vi "TriggererBoolean.vi"(8 "Boolean":bool, 10 "Control Name":string="Acquire Trigger", 11 "name or relative path":string="SW-Microscoper.vi") -> (0 "error out":errorcluster, 3 "VI out":refnum<vi>)   [LabVIEW 2012]
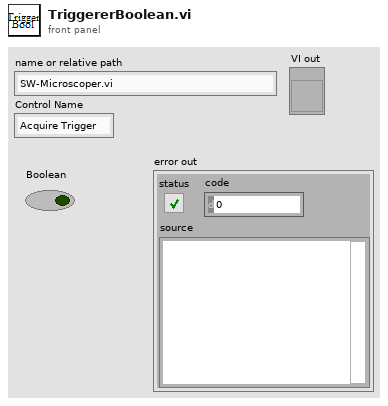
[diagram p1: front panel]
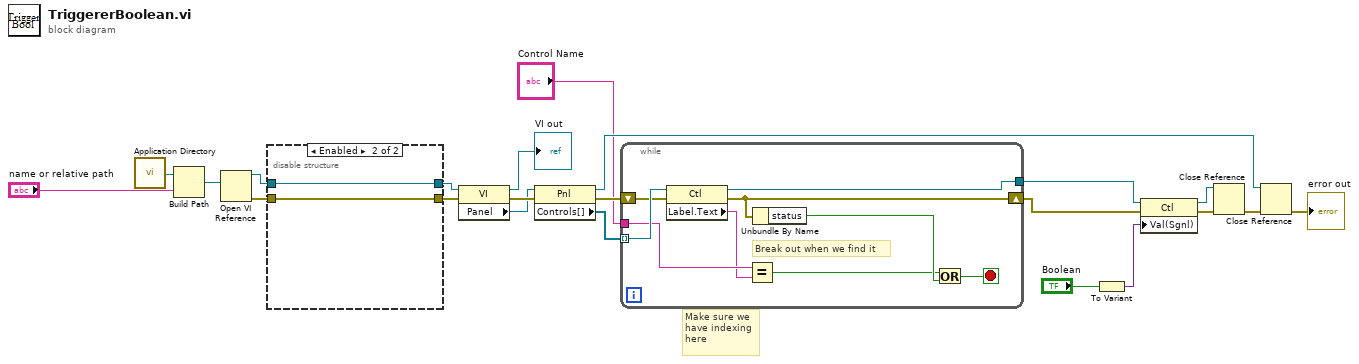
[diagram p0: block diagram]
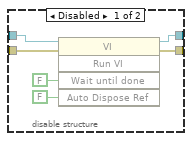
[diagram p2: hidden frame]
diagram:
  # "Make sure we\nhave indexing\nhere"
  n1 = call <vilib>:"Application Directory.vi"() -> ("Application Directory"=w10:path)
  n2 = Build Path(base path=w10, name or relative path="name or relative path") -> (appended path=w9:path)
  n3 = Open VI Reference(vi path=w9) -> (vi reference=w8:refnum<vi>, error out=w7:errorcluster)  [unwired: 5 in]
  n4 = disable-structure shown="Enabled" {
    disable-tunnel: w8 -> [w26 w30]
    disable-tunnel: w7 -> [w25 w29]
    disable-tunnel: [w24 w30] -> w6
    disable-tunnel: [w23 w29] -> w5
    frame Disabled {
      n5 = invoke class="VI" method="Run VI"(reference=w26, error in=w25, "Wait until done"=FALSE ("Front Panel Window:Open"), "Auto Dispose Ref"=FALSE ("Auto Dispose Reference")) -> (reference out=w24:refnum<vi>, error out=w23:errorcluster)  [unwired: 1 in, 3 out]
    }
    frame Enabled {
    }
  }
  n6 = property class="VI"(reference=w6, error in=w5) -> (reference out=→"VI out":refnum<vi>, error out=w16:errorcluster, "Panel"=w12:refnum<vi>)
  n7 = property class="Pnl"(reference=w12, error in=w16) -> (reference out=w22:refnum<vi>, error out=w17:errorcluster, "Controls[]"=w13:refnum<vi>[])
  n8 = while {
    tunnel: w13 -> [w39] mode=indexing
    tunnel: "Control Name" -> [w38]
    tunnel: [w36] -> w2
    shift-right: [w34] -> w1
    shift-left: w17 -> [w35]
    stop <- w33 stop-if-true
    # "Break out when we find it"
    n9 = property class="Ctl"(reference=w39, error in=w35) -> (reference out=w36:refnum<vi>, error out=w34:errorcluster, "Label.Text"=w37:string)
    n10 = Equal?(x=w38, y=w37) -> (x = y?=w31:bool)
    n11 = Unbundle By Name(w34) -> ("status"=w32:bool)
    n12 = Or(x=w31, y=w32) -> (x .or. y?=w33:bool)
  }
  n13 = To Variant(anything="Boolean") -> (Variant=w14:variant)
  n14 = property class="Ctl"(reference=w2, error in=w1, "Val(Sgnl)"=w14) -> (reference out=w21:refnum<vi>, error out=w20:errorcluster)
  n15 = Close Reference(reference=w21, error in (no error)=w20) -> (error out=w18:errorcluster)
  n16 = Close Reference(reference=w22, error in (no error)=w18) -> (error out=→"error out":errorcluster)
